vi "Acquire CPU load.vi"(8 "error in (no error)":errorcluster) -> (0 "error out":errorcluster, 2 "CPU load":u32)   [LabVIEW 2023, in "Acquisition.lvlib"]
doc: "Acquire CPU load."
uses:
  Acquisition.lvlib
  <resource>/objmgr/nisysapi.rc
  <resource>/objmgr/nicontrollersysapi.rc
  <vilib>/nisyscfg/nisyscfg.lvlib
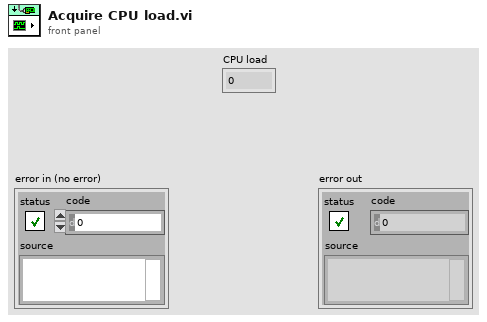
[diagram p1: front panel]
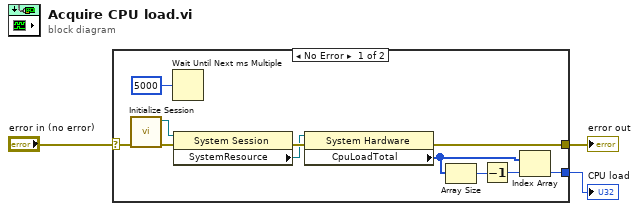
[diagram p0: block diagram]
diagram:
  n1 = case shown="No Error" "error in (no error)" {
    selector: "error in (no error)" -> [w13 w15]
    tunnel: [w4 w15] -> w2
    tunnel: [w5 _] -> w1
    frame No Error {
      n2 = call <vilib>:"Initialize Session.vi"("error in (no error)"=w13) -> ("error out"=w12:errorcluster, "Session out"=w9:refnum<k21>)  [unwired: 9 in]
      n3 = Wait Until Next ms Multiple(millisecond multiple=u32 5000) -> ()  [unwired: 1 out]
      n4 = property class="System Session"(reference=w9, error in=w12) -> (error out=w11:errorcluster, "SystemResource"=w10:refnum<k20>)  [unwired: 1 out]
      n5 = property class="System Hardware"(reference=w10, error in=w11) -> (error out=w4:errorcluster, "CpuLoadTotal"=w8:u32[])  [unwired: 1 out]
      n6 = Array Size(array=w8) -> (size(s)=w7:i32)
      n7 = Decrement(x=w7) -> (x-1=w6:i32)
      n8 = Index Array(array=w8, index=w6) -> (element=w5:u32)
    }
    frame Error {
    }
  }
  "error out" <- w2
  "CPU load" <- w1
